vi "Destroy.vi"(8 "error in (no error)":errorcluster, 11 "Stop Loop in":refnum<class "Parallel.lvclass">) -> (0 "error out":errorcluster)   [LabVIEW 2020, in "Test Executive.lvlib" / "Parallel.lvclass"]
uses:
  <vilib>/gpm_packages/@cs/test-executive/Source/Test Executive/Parallel/Parallel.lvclass
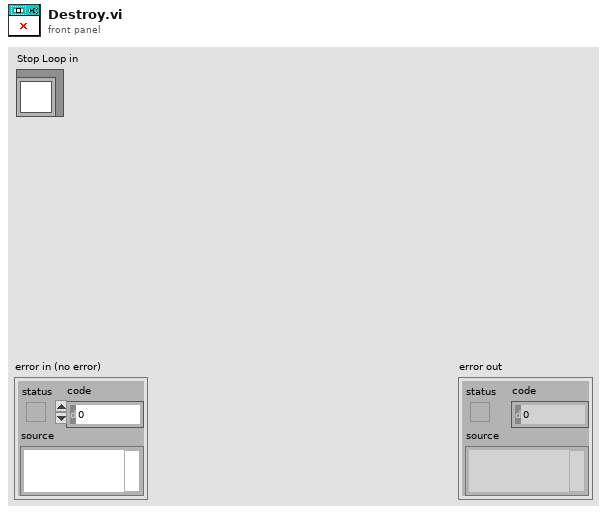
[diagram p1: front panel]
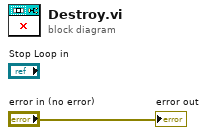
[diagram p0: block diagram]
diagram:
  "error out" <- "error in (no error)"
